vi "Get Harm(SubVI).vi"(8 "错误输入（无错误）":errorcluster, 11 "VISA引用句柄输入":refnum<visa-resource-name>) -> (0 "错误输出":errorcluster, 1 "harm":string, 3 "VISA引用句柄输出":refnum<visa-resource-name>)   [LabVIEW 2019, in "SubVI.lvlib"]
uses:
  SubVI.lvlib
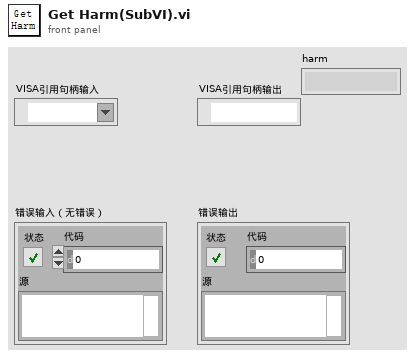
[diagram p1: front panel]
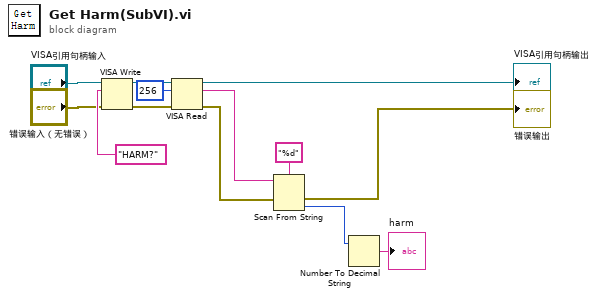
[diagram p0: block diagram]
diagram:
  n1 = VISA Write(VISA resource name="VISA引用句柄输入", write buffer="HARM?" ("format string"), error in (no error)="错误输入（无错误）") -> (VISA resource name out=w6:refnum<visa-resource-name>, error out=w7:errorcluster)  [unwired: 1 out]
  n2 = VISA Read(VISA resource name=w6, byte count=u32 256, error in (no error)=w7) -> (VISA resource name out=→"VISA引用句柄输出":refnum<visa-resource-name>, read buffer=w11:string, error out=w9:errorcluster)  [unwired: 1 out]
  n3 = Scan From String(format string="%d", input string=w11, error in=w9) -> (error out=→"错误输出":errorcluster, output 1=w2:i32)  [unwired: 2 in, 2 out]
  n4 = Number To Decimal String(number=w2) -> (decimal integer string=→"harm":string)  [unwired: 1 in]
